vi "FRCts20_Backend_CompetitionRoot_GET_reform.vi"(8 "error in (no error)":errorcluster, 11 "recordset data":variant[][](array[variant])) -> (0 "error out":errorcluster, 3 "data string":string)   [LabVIEW 2014]
uses:
  <vilib>/addons/database/_DB Variant To Data/Database Variant To Data.xnode
  FRCts20_Backend_Engine.lvlib
  FRCts20_Backend_API/FRCts20_Backend_API_CompetitionRoot.ctl
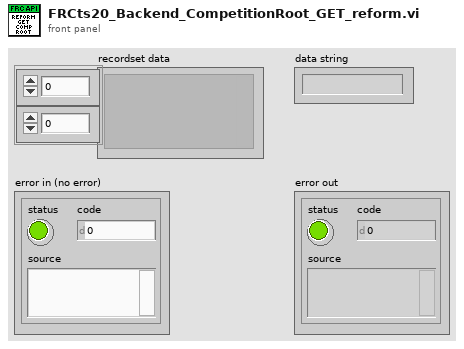
[diagram p1: front panel]
types:
  T1 = typedef "FRCts20_Backend_API.lvlib/FRCts20_Backend_API_CompetitionRoot.ctl" = cluster{"Competitions":string[], "APIReturn":string}
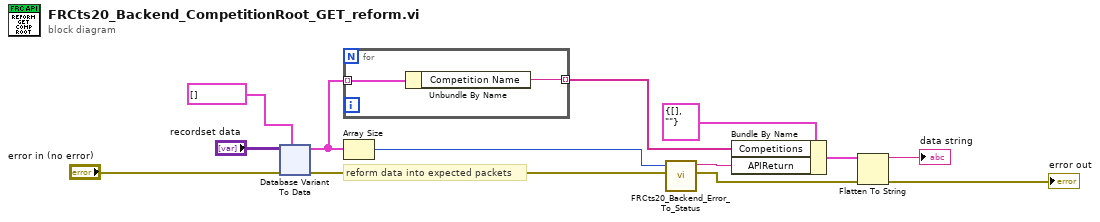
[diagram p0: block diagram]
diagram:
  # "reform data into expected packets"
  n1 = xnode "Database Variant To Data"("database variant"="recordset data", "error in"="error in (no error)", "type"=cluster{"Competition Name":string}[] []) -> ("data"=w3:cluster{"Competition Name":string}[], "error out"=w5:errorcluster)
  n2 = for {
    tunnel: w3 -> [w15] mode=indexing
    tunnel: [w14] -> w6 mode=indexing
    n3 = Unbundle By Name(w15) -> ("Competition Name"=w14:string)
  }
  n4 = Array Size(array=w3) -> (size(s)=w7:i32)
  n5 = call "FRCts20_Backend_Error_To_Status.vi"("error in (no error)"=w5, "rows affected"=w7) -> ("error out"=w8:errorcluster, "String"=w10:string)  [unwired: 8 in]
  n6 = Bundle By Name(cluster=T1 {"Competitions"=[], "APIReturn"=""} ("Competitions"), "Competitions"=w6, "APIReturn"=w10) -> (w11:T1)
  n7 = Flatten To String(anything=w11, error in (no error)=w8) -> (data string=→"data string":string, error out=→"error out":errorcluster)  [unwired: 2 in, 1 out]
